vi "(TestVI)DW7802 PWL UI Test.vi"() -> ()   [LabVIEW 2020]
uses:
  <vilib>/Utility/miscctls.llb/LVPoint32TypeDef.ctl
  <vilib>/Utility/miscctls.llb/LVPositionTypeDef.ctl
  <vilib>/Utility/miscctls.llb/LVBoundsTypeDef.ctl
  <vilib>/Utility/miscctls.llb/LVRowAndColumnTypeDef.ctl
panel:
  in  "Ramp 2":u16(ring) items=["Step", "Ramp (Lin)", "Ramp (exp)"]
  in  "버튼":bool
  out "선택 크기[]":u32[](array[numeric])
  out "선택 시작[]":u32[](array[numeric])
  out "경계":T1
  out "위치":T2
  out "좌표":T3
  in  "배열 3":T4(array[cluster]) {"Frequency" min=40.0 max=300.0 step=1.0; "Cycle" items=["0.5"=0.5, "1"=1.0, "1.5"=1.5, "2"=2.0, "2.5"=2.5, "3"=3.0, "3.5"=3.5, "4"=4.0, "4.5"=4.5, "5"=5.0, "5.5"=5.5, "6"=6.0, "6.5"=6.5, "7"=7.0, "7.5"=7.5, "8"=8.0, "8.5"=8.5, "9"=9.0, "9.5"=9.5, "10"=10.0, "10.5"=10.5, "11"=11.0, "11.5"=11.5, "12"=12.0, "12.5"=12.5, "13"=13.0, "13.5"=13.5, "14"=14.0, "14.5"=14.5, "15"=15.0, "15.5"=15.5, "16"=16.0, "16.5"=16.5, "17"=17.0, "17.5"=17.5, "18"=18.0, "18.5"=18.5, "19"=19.0, "19.5"=19.5, "20"=20.0, "20.5"=20.5, "21"=21.0, "21.5"=21.5, "22"=22.0, "22.5"=22.5, "23"=23.0, "23.5"=23.5, "24"=24.0, "24.5"=24.5, "25"=25.0, "25.5"=25.5, "26"=26.0, "26.5"=26.5, "27"=27.0, "27.5"=27.5, "28"=28.0, "28.5"=28.5, "29"=29.0, "29.5"=29.5, "30"=30.0, "30.5"=30.5, "31"=31.0, "31.5"=31.5, "32"=32.0, "32.5"=32.5, "33"=33.0, "33.5"=33.5, "34"=34.0, "34.5"=34.5, "35"=35.0, "35.5"=35.5, "36"=36.0, "36.5"=36.5, "37"=37.0, "37.5"=37.5, "38"=38.0, "38.5"=38.5, "39"=39.0, "39.5"=39.5, "40"=40.0, "40.5"=40.5, "41"=41.0, "41.5"=41.5, "42"=42.0, "42.5"=42.5, "43"=43.0, "43.5"=43.5, "44"=44.0, "44.5"=44.5, "45"=45.0, "45.5"=45.5, "46"=46.0, "46.5"=46.5, "47"=47.0, "47.5"=47.5, "48"=48.0, "48.5"=48.5, "49"=49.0, "49.5"=49.5, "50"=50.0, "50.5"=50.5, "51"=51.0, "51.5"=51.5, "52"=52.0, "52.5"=52.5, "53"=53.0, "53.5"=53.5, "54"=54.0, "54.5"=54.5, "55"=55.0, "55.5"=55.5, "56"=56.0, "56.5"=56.5, "57"=57.0, "57.5"=57.5, "58"=58.0, "58.5"=58.5, "59"=59.0, "59.5"=59.5, "60"=60.0, "60.5"=60.5, "61"=61.0, "61.5"=61.5, "62"=62.0, "62.5"=62.5, "63"=63.0, "63.5"=63.5, "64"=64.0, "64.5"=64.5, "65"=65.0, "65.5"=65.5, "66"=66.0, "66.5"=66.5, "67"=67.0, "67.5"=67.5, "68"=68.0, "68.5"=68.5, "69"=69.0, "69.5"=69.5, "70"=70.0, "70.5"=70.5, "71"=71.0, "71.5"=71.5, "72"=72.0, "72.5"=72.5, "73"=73.0, "73.5"=73.5, "74"=74.0, "74.5"=74.5, "75"=75.0, "75.5"=75.5, "76"=76.0, "76.5"=76.5, "77"=77.0, "77.5"=77.5, "78"=78.0, "78.5"=78.5, "79"=79.0, "79.5"=79.5, "80"=80.0, "80.5"=80.5, "81"=81.0, "81.5"=81.5, "82"=82.0, "82.5"=82.5, "83"=83.0, "83.5"=83.5, "84"=84.0, "84.5"=84.5, "85"=85.0, "85.5"=85.5, "86"=86.0, "86.5"=86.5, "87"=87.0, "87.5"=87.5, "88"=88.0, "88.5"=88.5, "89"=89.0, "89.5"=89.5, "90"=90.0, "90.5"=90.5, "91"=91.0, "91.5"=91.5, "92"=92.0, "92.5"=92.5, "93"=93.0, "93.5"=93.5, "94"=94.0, "94.5"=94.5, "95"=95.0, "95.5"=95.5, "96"=96.0, "96.5"=96.5, "97"=97.0, "97.5"=97.5, "98"=98.0, "98.5"=98.5, "99"=99.0, "99.5"=99.5, "100"=100.0, "100.5"=100.5, "101"=101.0, "101.5"=101.5, "102"=102.0, "102.5"=102.5, "103"=103.0, "103.5"=103.5, "104"=104.0, "104.5"=104.5, "105"=105.0, "105.5"=105.5, "106"=106.0, "106.5"=106.5, "107"=107.0, "107.5"=107.5, "108"=108.0, "108.5"=108.5, "109"=109.0, "109.5"=109.5, "110"=110.0, "110.5"=110.5, "111"=111.0, "111.5"=111.5, "112"=112.0, "112.5"=112.5, "113"=113.0, "113.5"=113.5, "114"=114.0, "114.5"=114.5, "115"=115.0, "115.5"=115.5, "116"=116.0, "116.5"=116.5, "117"=117.0, "117.5"=117.5, "118"=118.0, "118.5"=118.5, "119"=119.0, "119.5"=119.5, "120"=120.0, "120.5"=120.5, "121"=121.0, "121.5"=121.5, "122"=122.0, "122.5"=122.5, "123"=123.0, "123.5"=123.5, "124"=124.0, "124.5"=124.5, "125"=125.0, "125.5"=125.5, "126"=126.0, "126.5"=126.5, "127"=127.0, "127.5"=127.5]; "Amplitude" items=["0"=0.0, "10"=0.1, "20"=0.2, "30"=0.3, "40"=0.4, "50"=0.5, "60"=0.6, "70"=0.7, "80"=0.8, "90"=0.9, "100"=1.0]; "Ramp 4" items=["Step"=0, "Ramp (Lin.)"=1, "Ramp (Exp.)"=3]; "Shape" items=["Sine", "Square"]}
  in  "WF Seq 3":i32[](listbox)
  in  "Ramp":u16(ring) items=["Step", "Ramp - Lin.", "Ramp - Exp."]
  in  "배열 2":T5(array[cluster]) {"Cycle" items=["0.5", "1", "1.5", "2", "2.5", "3", "3.5", "4", "4.5", "5", "5.5", "6", "6.5", "7", "7.5", "8", "8.5", "9", "9.5", "10", "10.5", "11", "11.5", "12", "12.5", "13", "13.5", "14", "14.5", "15", "15.5", "16", "16.5", "17", "17.5", "18", "18.5", "19", "19.5", "20", "20.5", "21", "21.5", "22", "22.5", "23", "23.5", "24", "24.5", "25"]; "Amplitude" items=["0", "10", "20", "30", "40", "50", "60", "70", "80", "90", "100"]; "Ramp Type" items=["Lin.", "Exp.", ""]; "Ramp" items=["Step", "Ramp"]; "Shape" items=["Sine", "Square"]}
  in  "배열":T6(array[cluster]) {"Shape 5" items=["0", "1", "2", "3", "4", "5", "6", "7"]; "Shape 4" items=["0", "10", "20", "30", "40", "50", "60", "70", "80", "90", "100"]; "Shape 3" items=["Lin.", "Exp."]; "Shape 2" items=["Step", "Ramp"]; "Shape" items=["Sine", "Square"]}
  in  "WF Seq 2":i32[](listbox)
  in  "텍스트 링":u16(ring) items=["Sine", "Square"]
  in  "텍스트 링 2":u16(ring) items=["Sine", "Square"]
  in  "클러스터 2":T7 {"클러스터 7"."Shape 5" items=["0", "1", "2", "3", "4", "5", "6", "7"]; "클러스터 7"."Shape 4" items=["0", "10", "20", "30", "40", "50", "60", "70", "80", "90", "100"]; "클러스터 7"."Shape 3" items=["Lin.", "Exp."]; "클러스터 7"."Shape 2" items=["Step", "Ramp"]; "클러스터 7"."Shape" items=["Sine", "Square"]; "클러스터 6"."Shape 5" items=["0", "1", "2", "3", "4", "5", "6", "7"]; "클러스터 6"."Shape 4" items=["0", "10", "20", "30", "40", "50", "60", "70", "80", "90", "100"]; "클러스터 6"."Shape 3" items=["Lin.", "Exp."]; "클러스터 6"."Shape 2" items=["Step", "Ramp"]; "클러스터 6"."Shape" items=["Sine", "Square"]; "클러스터 5"."Shape 5" items=["0", "1", "2", "3", "4", "5", "6", "7"]; "클러스터 5"."Shape 4" items=["0", "10", "20", "30", "40", "50", "60", "70", "80", "90", "100"]; "클러스터 5"."Shape 3" items=["Lin.", "Exp."]; "클러스터 5"."Shape 2" items=["Step", "Ramp"]; "클러스터 5"."Shape" items=["Sine", "Square"]; "클러스터 4"."Shape 5" items=["0", "1", "2", "3", "4", "5", "6", "7"]; "클러스터 4"."Shape 4" items=["0", "10", "20", "30", "40", "50", "60", "70", "80", "90", "100"]; "클러스터 4"."Shape 3" items=["Lin.", "Exp."]; "클러스터 4"."Shape 2" items=["Step", "Ramp"]; "클러스터 4"."Shape" items=["Sine", "Square"]; "클러스터 3"."Shape 5" items=["0", "1", "2", "3", "4", "5", "6", "7"]; "클러스터 3"."Shape 4" items=["0", "10", "20", "30", "40", "50", "60", "70", "80", "90", "100"]; "클러스터 3"."Shape 3" items=["Lin.", "Exp."]; "클러스터 3"."Shape 2" items=["Step", "Ramp"]; "클러스터 3"."Shape" items=["Sine", "Square"]; "클러스터 2"."Shape 5" items=["0", "1", "2", "3", "4", "5", "6", "7"]; "클러스터 2"."Shape 4" items=["0", "10", "20", "30", "40", "50", "60", "70", "80", "90", "100"]; "클러스터 2"."Shape 3" items=["Lin.", "Exp."]; "클러스터 2"."Shape 2" items=["Step", "Ramp"]; "클러스터 2"."Shape" items=["Sine", "Square"]; "클러스터"."Shape 5" items=["0", "1", "2", "3", "4", "5", "6", "7"]; "클러스터"."Shape 4" items=["0", "10", "20", "30", "40", "50", "60", "70", "80", "90", "100"]; "클러스터"."Shape 3" items=["Lin.", "Exp."]; "클러스터"."Shape 2" items=["Step", "Ramp"]; "클러스터"."Shape" items=["Sine", "Square"]}
  in  "클러스터":T8 {"Shape 5" items=["0", "1", "2", "3", "4", "5", "6", "7"]; "Shape 4" items=["0", "10", "20", "30", "40", "50", "60", "70", "80", "90", "100"]; "Shape 3" items=["Lin.", "Exp."]; "Shape 2" items=["Step", "Ramp"]; "Shape" items=["Sine", "Square"]}
  in  "정지":bool
  in  "WF Seq":i32[](listbox)
  # "위로 네칸\n오른쪽으로 두칸"
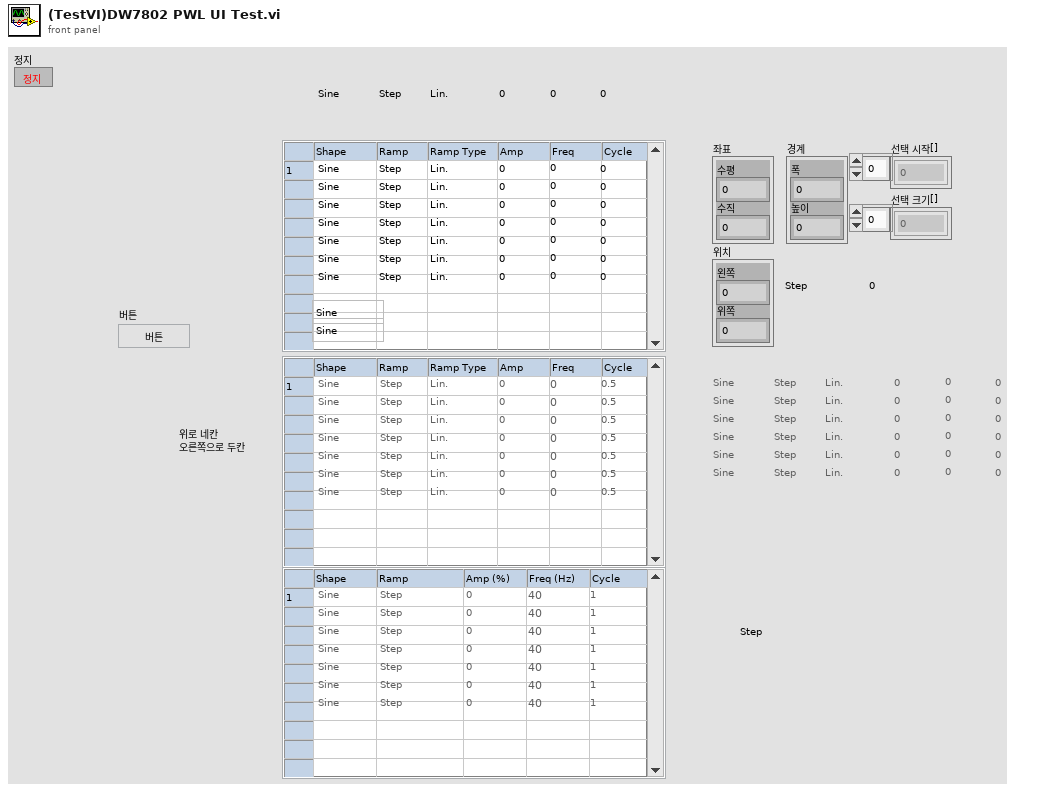
[diagram p1: front panel]
types:
  T1 = typedef "LVBoundsTypeDef.ctl" = cluster{"Width":u32, "Height":u32}
  T2 = typedef "LVPositionTypeDef.ctl" = cluster{"Left":i32, "Top":i32}
  T3 = typedef "LVPoint32TypeDef.ctl" = cluster{"Horizontal":i32, "Vertical":i32}
  T4 = cluster{"Shape":u16, "Ramp 4":u16, "Amplitude":dbl, "Frequency":dbl, "Cycle":dbl}[]
  T5 = cluster{"Shape":u16, "Ramp":u16, "Ramp Type":u16, "Amplitude":u16, "Frequency":dbl, "Cycle":u16}[]
  T6 = cluster{"Shape":u16, "Shape 2":u16, "Shape 3":u16, "Shape 4":u16, "Freq":u16, "Shape 5":u16}[]
  T7 = cluster{"클러스터":cluster{"Shape":u16, "Shape 2":u16, "Shape 3":u16, "Shape 4":u16, "Freq":u16, "Shape 5":u16}, "클러스터 2":cluster{"Shape":u16, "Shape 2":u16, "Shape 3":u16, "Shape 4":u16, "Freq":u16, "Shape 5":u16}, "클러스터 3":cluster{"Shape":u16, "Shape 2":u16, "Shape 3":u16, "Shape 4":u16, "Freq":u16, "Shape 5":u16}, "클러스터 4":cluster{"Shape":u16, "Shape 2":u16, "Shape 3":u16, "Shape 4":u16, "Freq":u16, "Shape 5":u16}, "클러스터 5":cluster{"Shape":u16, "Shape 2":u16, "Shape 3":u16, "Shape 4":u16, "Freq":u16, "Shape 5":u16}, "클러스터 6":cluster{"Shape":u16, "Shape 2":u16, "Shape 3":u16, "Shape 4":u16, "Freq":u16, "Shape 5":u16}, "클러스터 7":cluster{"Shape":u16, "Shape 2":u16, "Shape 3":u16, "Shape 4":u16, "Freq":u16, "Shape 5":u16}}
  T8 = cluster{"Shape":u16, "Shape 2":u16, "Shape 3":u16, "Shape 4":u16, "Freq":u16, "Shape 5":u16}
  T9 = typedef "LVRowAndColumnTypeDef.ctl" = cluster{"Row":i32, "Column":i32}
  T10 = cluster{"Shape":u16, "Ramp":u16, "Ramp Type":u16, "Amplitude":u16, "Frequency":dbl, "Cycle":u16}
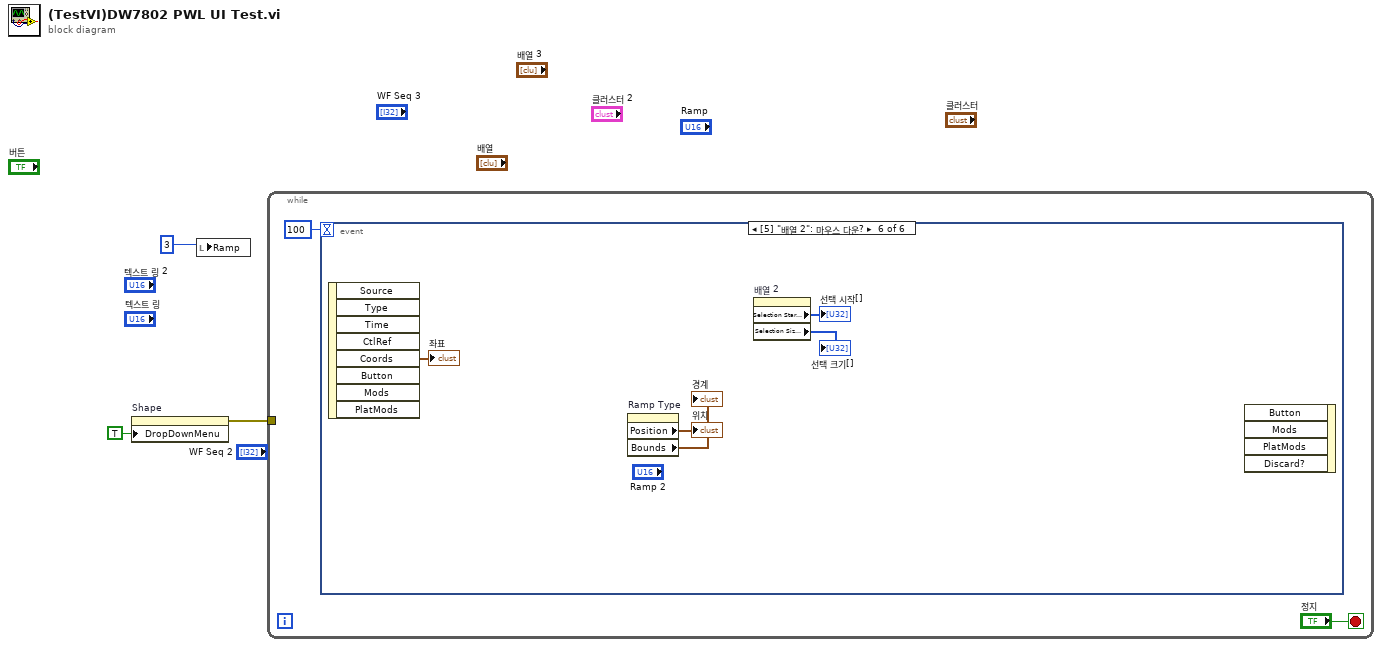
[diagram p0: block diagram]
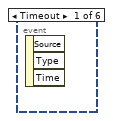
[diagram p2: hidden frame]
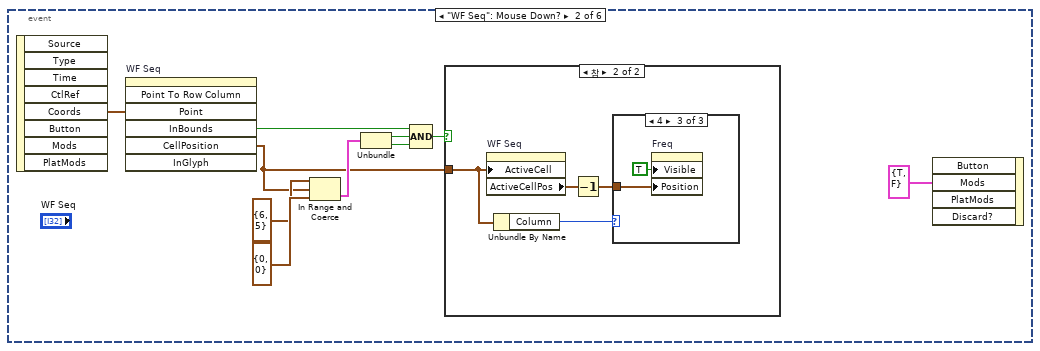
[diagram p3: hidden frame]
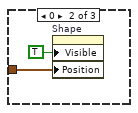
[diagram p6: hidden frame]
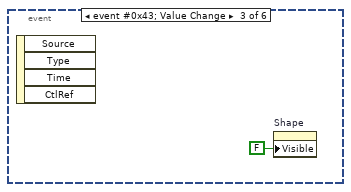
[diagram p7: hidden frame]
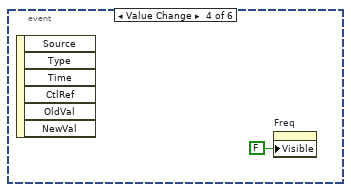
[diagram p8: hidden frame]
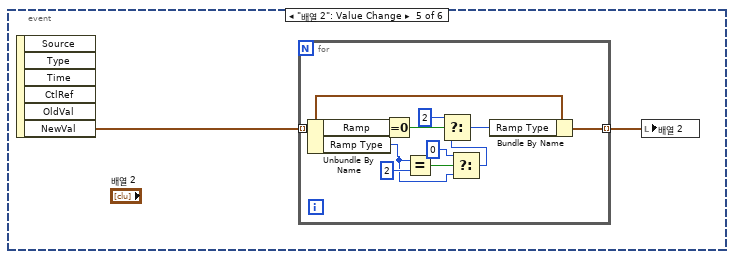
[diagram p9: hidden frame]
diagram:
  n1 = property on="Shape" class="Ring (엄격한)"("DropDownMenu"=TRUE ("Drop Down Menu")) -> (error out=w2:errorcluster)  [unwired: 2 in, 1 out]
  n2 = local write "Ramp"(u16 3) -> ()
  n3 = while {
    tunnel: w2 -> [_]
    stop <- "정지" stop-if-true
    n4 = event shown="[5] \"배열 2\": 마우스 다운?" {
      selector: _ -> [_ _ _ _ _ _]
      dyn-events: _ -> [_ _ _ _ _ _]
      timeout: 100 -> [_ _ _ _ _ _]
      event Timeout {
        n5 = event-data() -> ()  [unwired: 1 in, 3 out]
      }
      event "WF Seq": Mouse Down? {
        n6 = event-data() -> ("Coords"=w15:T3)  [unwired: 1 in, 7 out]
        n7 = invoke on="WF Seq" class="MCListbox (엄격한)" method="Point To Row Column"("Point"=w15) -> ("InBounds"=w14:bool, "CellPosition"=w7:T9)  [unwired: 6 in, 5 out]
        n8 = In Range and Coerce(upper limit=T9 {"Row"=6, "Column"=5} ("상위 리미트"), x=w7, lower limit=T9 {"Row"=0, "Column"=0} ("하위 리미트")) -> (In Range?=w11:cluster{"Row":bool, "Column":bool})  [unwired: 1 out]
        n9 = Unbundle(w11) -> ("Row"=w10:bool, "Column"=w9:bool)
        n10 = Compound Arithmetic op=AND(w14, w10, w9) -> (w8:bool)
        n11 = case shown="참" w8 {
          tunnel: w7 -> [_ w17]
          frame False {
          }
          frame True {
            n12 = property on="WF Seq" class="MCListbox (엄격한)"("ActiveCell"=w17) -> ("ActiveCellPos"=w18:T2)  [unwired: 2 in, 2 out]
            n13 = Unbundle By Name(w17) -> ("Column"=w16:i32)
            n14 = Decrement(x=w18) -> (x-1=w19:T2)
            n15 = case shown="4" w16 {
              tunnel: w19 -> [_ w21 w23]
              frame Default {
              }
              frame 0 {
                n16 = property on="Shape" class="Ring (엄격한)"("Visible"=TRUE ("보이기"), "Position"=w21) -> ()  [unwired: 2 in, 2 out]
              }
              frame 4 {
                n17 = property on="Freq" class="DigNum (엄격한)"("Visible"=TRUE ("보이기"), "Position"=w23) -> ()  [unwired: 2 in, 2 out]
              }
            }
          }
        }
        n18 = event-data("Mods"=cluster{"Double Click":bool, "Menu Key":bool} {"Double Click"=TRUE, "Menu Key"=FALSE} ("조합키")) -> ()  [unwired: 4 in, 1 out]
      }
      event "클러스터.Shape": event #0x43; "클러스터.Shape": Value Change {
        n19 = event-data() -> ()  [unwired: 1 in, 4 out]
        n20 = property on="Shape" class="Ring (엄격한)"("Visible"=FALSE ("보이기")) -> ()  [unwired: 2 in, 2 out]
      }
      event "클러스터.Freq": Value Change {
        n21 = event-data() -> ()  [unwired: 1 in, 6 out]
        n22 = property on="Freq" class="DigNum (엄격한)"("Visible"=FALSE ("보이기")) -> ()  [unwired: 2 in, 2 out]
      }
      event "배열 2": Value Change {
        n23 = event-data() -> ("NewVal"=w27:T5)  [unwired: 1 in, 5 out]
        n24 = for {
          tunnel: w27 -> [w38] mode=indexing
          tunnel: [w33] -> w26 mode=indexing
          n25 = Unbundle By Name(w38) -> ("Ramp"=w37:u16, "Ramp Type"=w29:u16)
          n26 = Equal To 0?(x=w37) -> (x = 0?=w36:bool)
          n27 = Equal?(x=w29, y=u16 2) -> (x = y?=w31:bool)
          n28 = Select(t=u16 0 ("y"), s=w31, f=w29) -> (s? t:f=w28:u16)
          n29 = Select(t=u16 2 ("Ramp Type"), s=w36, f=w28) -> (s? t:f=w34:u16)
          n30 = Bundle By Name(cluster=w38, "Ramp Type"=w34) -> (w33:T10)
        }
        n31 = local write "배열 2"(w26) -> ()
      }
      event "배열 2": Mouse Down? {
        n32 = event-data() -> ("Coords"=→"좌표":T3)  [unwired: 1 in, 7 out]
        n33 = property on="Ramp Type" class="Ring (엄격한)"() -> ("Position"=→"위치":T2, "Bounds"=→"경계":T1)  [unwired: 2 in, 2 out]
        n34 = property on="배열 2" class="Arr (엄격한)"() -> ("Selection Start []"=→"선택 시작[]":u32[], "Selection Size []"=→"선택 크기[]":u32[])  [unwired: 2 in, 2 out]
        n35 = event-data() -> ()  [unwired: 5 in, 1 out]
      }
    }
  }
